vi "st_Discrete Uniform PDF (kx).vi"(10 "n":i32=100, 11 "x":dbl=1.0) -> (0 "error":i32, 3 "pdf(x)":dbl=0.01)   [LabVIEW 2010, in "NI_Gmath.lvlib"]
uses:
  NI_Gmath.lvlib
  st_error_code.ctl
panel:
  # "Discrete Uniform PDF (kx)"
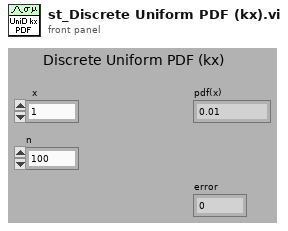
[diagram p1: front panel]
types:
  T1 = typedef "NI_Gmath.lvlib/st_error_code.ctl" = i32
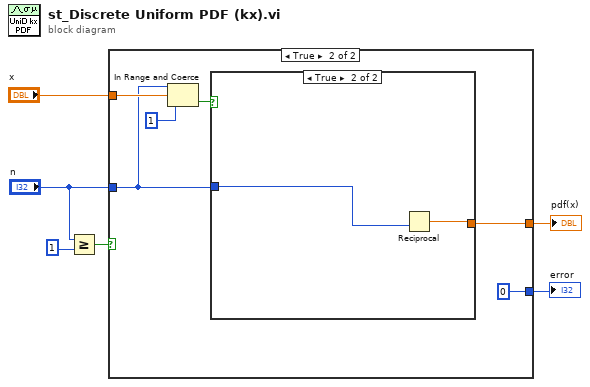
[diagram p0: block diagram]
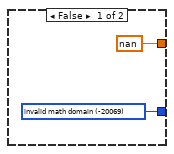
[diagram p2: hidden frame]
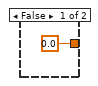
[diagram p3: hidden frame]
diagram:
  n1 = Greater Or Equal?(x="n", y=1) -> (x >= y?=w1:bool)
  n2 = case shown="True" w1 {
    tunnel: [w8 0 ("invalid math domain")] -> w6
    tunnel: [nan w10] -> w5
    tunnel: "x" -> [_ w12]
    tunnel: "n" -> [_ w11]
    frame False {
      w8 = T1 -20069 items=["invalid math domain"=-20069, "Fourier interpolation size m >= n"=-20070, "empty array"=-20003] ("stat interp error code")
    }
    frame True {
      n3 = In Range and Coerce(upper limit=w11, x=w12, lower limit=1) -> (In Range?=w9:bool)  [unwired: 1 out]
      n4 = case shown="True" w9 {
        tunnel: [0.0 w16] -> w10
        tunnel: w11 -> [_ w17]
        frame False {
        }
        frame True {
          n5 = Reciprocal(x=w17) -> (1/x=w16:dbl)
        }
      }
    }
  }
  "pdf(x)" <- w5
  "error" <- w6
